vi "Call JSON.vi"(4 "ArgumentsKw":string, 6 "Arguments":string, 7 "Options":string, 8 "Error in":errorcluster, 9 "Timeout (ms)":i32=500, 10 "Topic URI":string, 11 "WAMP Client in":refnum<class "WAMP Client.lvclass">) -> (0 "Error out":errorcluster, 1 "ArgumentKw Payload":string, 2 "Arguments Payload":string, 3 "WAMP Client out":refnum<class "WAMP Client.lvclass">, 5 "WAMP Error":T1={"URI"="", "Arguments Payload"="", "ArgumentKw Payload"="{}", "Details"="{}", "Associated LabVIEW Error"={"status"=FALSE, "code"=0, "source"=""}})   [LabVIEW 2020, in "wamplv.lvlib" / "WAMP Client.lvclass"]
uses:
  WAMP Client.lvclass
  WAMP Client.lvclass/WAMP Client.ctl
  7e7f57fc-00c7-4146-ad98-96717bb40580.vi
  Call (async) JSON.vi
  TypeDefs/Error or abort detail (JSON).ctl
  wamplv.lvlib
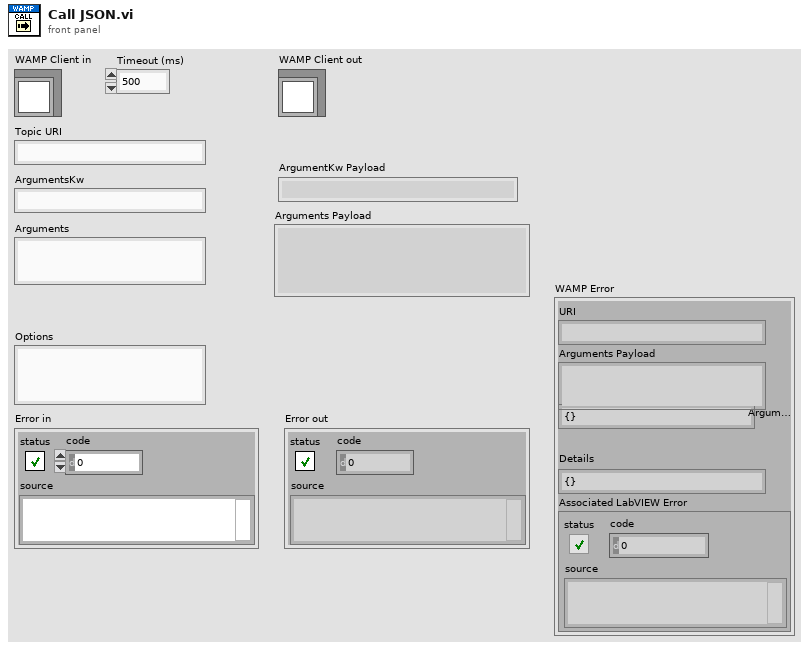
[diagram p1: front panel]
types:
  T1 = typedef "wamplv.lvlib/Error or abort detail (JSON).ctl" = cluster{"URI":string, "Arguments Payload":string, "ArgumentKw Payload":string, "Details":string, "Associated LabVIEW Error":errorcluster}
  T2 = typedef "wamplv.lvlib/WAMP Client.lvclass/RESULT payload (JSON).ctl" = cluster{"Topic":string, "Arguments Payload":string, "ArgumentKw Payload":string, "Details":string, "Error/Abort details (JSON)":T1}
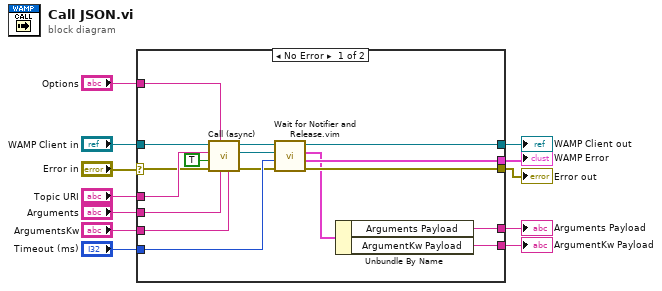
[diagram p0: block diagram]
diagram:
  n1 = case shown="No Error" "Error in" {
    selector: "Error in" -> [w24 w31]
    tunnel: [w22 w31] -> w11
    tunnel: [w17 w30] -> w9
    tunnel: "WAMP Client in" -> [w29 w30]
    tunnel: "Topic URI" -> [w26 _]
    tunnel: "Arguments" -> [w28 _]
    tunnel: "ArgumentsKw" -> [w27 _]
    tunnel: "Timeout (ms)" -> [w23 _]
    tunnel: [w21 _] -> w2
    tunnel: [w20 _] -> w4
    tunnel: "Options" -> [w25 _]
    tunnel: [w19 _] -> w1
    frame No Error {
      n2 = call-poly "Call (async).vi"("ArgumentsKw"=w27, "Arguments"=w28, "Options"=w25, "error in (no error)"=w24, "Notify result"=TRUE, "Topic URI"=w26, "WAMP Client in"=w29) -> ("error out"=w14:errorcluster, "Call result notifier"=w13:refnum<notifier>, "WAMP Client out"=w15:refnum<class "WAMP Client.lvclass">)  [unwired: 2 in]
      n3 = call "Wait for Notifier and Release.vim"("error in (no error)"=w14, "timeout in ms (0)"=w23, "Notifier in"=w13, "WAMP Client in"=w15) -> ("error out"=w22:errorcluster, "WAMP Error"=w19:T1, "Data"=w18:T2, "WAMP Client out"=w17:refnum<class "WAMP Client.lvclass">)  [unwired: 4 in]
      n4 = Unbundle By Name(w18) -> ("Arguments Payload"=w21:string, "ArgumentKw Payload"=w20:string)
    }
    frame Error {
    }
  }
  "Error out" <- w11
  "WAMP Client out" <- w9
  "Arguments Payload" <- w2
  "ArgumentKw Payload" <- w4
  "WAMP Error" <- w1
